vi "Remove Station Config Item.vi"(10 "Tag":T3, 11 "Station Config in":T2) -> (2 "map":map{i32, T1}(c390), 3 "Station Config out":T2)   [LabVIEW 2025, in "Full User Interface.lvlib"]
uses:
  Full User Interface.lvlib
  Station Config.ctl
  Station Info.ctl
  <vilib>/Utility/miscctls.llb/LVMapReplaceAction.ctl
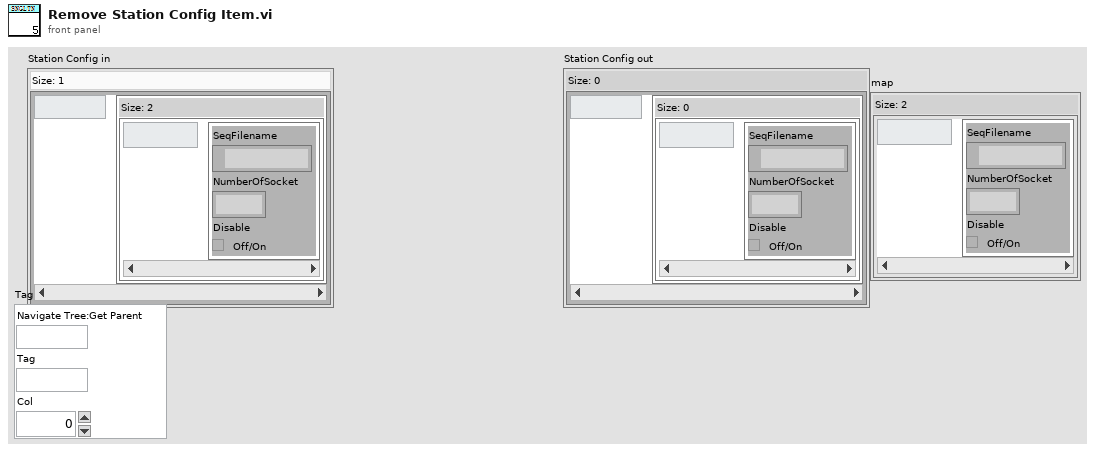
[diagram p1: front panel]
types:
  T1 = typedef "Full User Interface.lvlib/Station Info.ctl" = cluster{"SeqFilename":path, "NumberOfSocket":i32, "Disable":bool}
  T2 = typedef "Full User Interface.lvlib/Station Config.ctl" = map{string, map{i32, T1}}
  T3 = cluster{"Navigate Tree:Get Parent":string, "Tag":string, "Col":i32}
  T4 = typedef "LVMapReplaceAction.ctl" = enum32{"Modify Entry only if found", "Add or Modify Entry", "Delete Entry"}
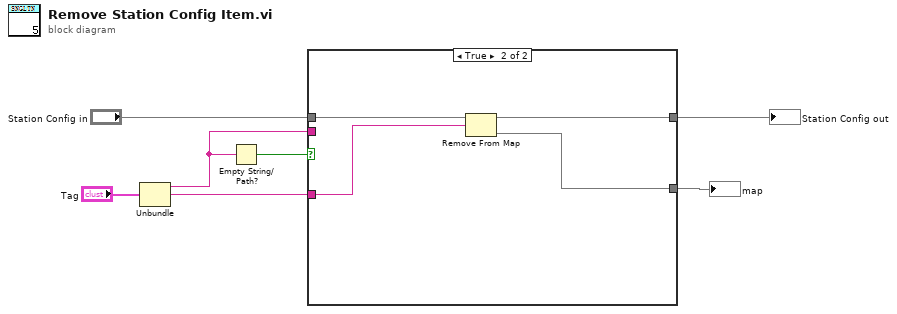
[diagram p0: block diagram]
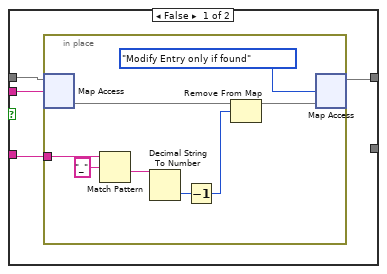
[diagram p2: hidden frame]
diagram:
  n1 = Unbundle("Tag") -> ("Navigate Tree:Get Parent"=w5:string, "Tag"=w3:string)  [unwired: 1 out]
  n2 = Empty String/Path?(string/path=w5) -> (empty?=w4:bool)
  n3 = case shown="True" w4 {
    tunnel: "Station Config in" -> [w10 w23]
    tunnel: w5 -> [w9 _]
    tunnel: [w8 w22] -> w2
    tunnel: w3 -> [w11 w21]
    tunnel: [_ w20] -> w1
    frame False {
      n4 = in-place {
        in-place-border: w11 -> [w17]
        n5 = in-place-map #1(w10, w9) -> (w15:map{i32, T1})  [unwired: 1 in, 1 out]
        n6 = Match Pattern(string=w17, regular expression="_") -> (after substring=w18:string)  [unwired: 1 in, 3 out]
        n7 = Decimal String To Number(string=w18) -> (number=w13:i32)  [unwired: 2 in, 1 out]
        n8 = Decrement(x=w13) -> (x-1=w12:i32)
        n9 = Remove From Map(10:w12, 11:w15) -> (3:w14:map{i32, T1})  [unwired: 2 out]
        n10 = in-place-map #1(w14, LVMapReplaceAction."Modify Entry only if found" ("action")) -> (w8:T2)  [unwired: 2 out]
      }
    }
    frame True {
      n11 = Remove From Map(10:w21, 11:w23) -> (1:w20:map{i32, T1}, 3:w22:T2)  [unwired: 1 out]
    }
  }
  "Station Config out" <- w2
  "map" <- w1
